vi "Filter Get Averaging Factor.vi"(11 "averagingFactor":i32) -> (2 "function return":u32, 3 "averagingFactor out":i32)   [LabVIEW 2018, in "AndorSDK.lvlib"]
doc: "EXPNETTYPE unsigned int WINAPI Filter_GetAveragingFactor(int * averagingFactor);"
uses:
  AndorSDK.lvlib
  ATMCD32D.dll
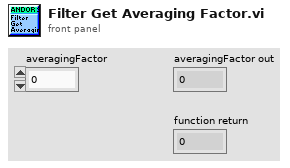
[diagram p1: front panel]
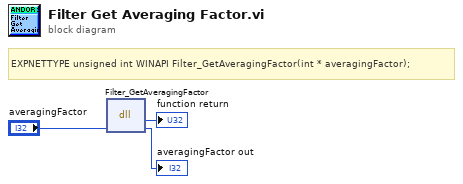
[diagram p0: block diagram]
diagram:
  # "EXPNETTYPE unsigned int WINAPI Filter_GetAveragingFactor(int * averagingFactor);"
  n1 = dll-call lib="PTH2babs E\nPersönliches02 - Arbeit03-HiwijobsLabviewCodelibANDOR\tAndor SDK\nATMCD32D.*" fn="Filter_GetAveragingFactor"("averagingFactor"="averagingFactor") -> (→"function return":u32, "averagingFactor"=→"averagingFactor out":i32)  [unwired: 3 in, 2 out]
